vi "reset_led.vi"(11 "Array":refnum<vi>[](array[refnum])) -> ()   [LabVIEW 2011]
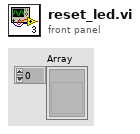
[diagram p1: front panel]
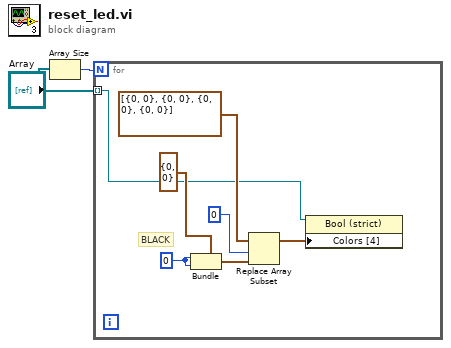
[diagram p0: block diagram]
diagram:
  n1 = Array Size(array="Array") -> (size(s)=w2:i32)
  n2 = for {
    N: w2 -> [_]
    tunnel: "Array" -> [w3] mode=indexing
    w4 = 0
    # "BLACK"
    n3 = Bundle(cluster=cluster{u32, u32} {0, 0}, w4, w4) -> (w7:cluster{u32, u32})
    n4 = Replace Array Subset(array=cluster{u32, u32}[] [{0, 0}, {0, 0}, {0, 0}, {0, 0}] ("Colors [4]"), new element=w7, index=0) -> (w9:cluster{u32, u32}[])
    n5 = property on="Property Node" class="Bool (strict)"(reference=w3, "Colors [4]"=w9) -> ()  [unwired: 1 in, 2 out]
  }
